vi "test_add_errors.vi"() -> ()   [LabVIEW 2020]
uses:
  <vilib>/Utility/miscctls.llb/LVPointTypeDef.ctl
panel:
  out "error out":errorcluster
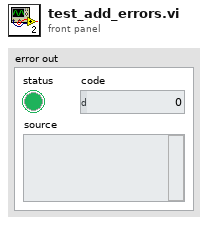
[diagram p1: front panel]
types:
  T1 = typedef "LVPointTypeDef.ctl" = cluster{"Horizontal":i16, "Vertical":i16}
  T2 = enum32{"invalid VI type", "Standard VI", "Control VI", "Global VI", "Polymorphic VI", "Configuration VI", "SubSystem", "Facade VI", "Method VI", "Statechart Diagram VI"}
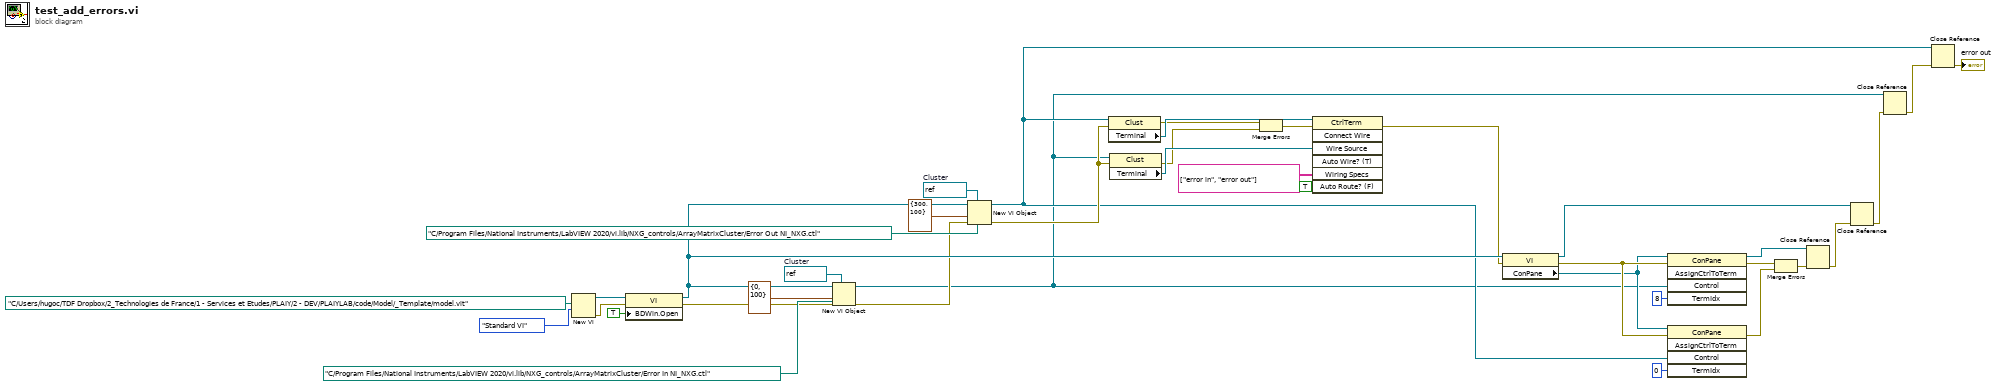
[diagram p0: block diagram]
diagram:
  w27 = refnum<vi> refnum  # Cluster
  w34 = refnum<vi> refnum  # Cluster
  n1 = New VI(9:T2."Standard VI" ("vi type (standard vi)"), 10:path "C:/Users/hugoc/TDF Dropbox/2_Technologies de France/1 - Services et Etudes/PLAIY/2 - DEV/PLAIYLAB/code/Model/_Template/model.vit" ("template")) -> (0:w36:errorcluster, 3:w30:refnum<vi>)  [unwired: 5 in]
  n2 = property class="VI"(reference=w30, error in=w36, "BDWin.Open"=TRUE ("Block Diagram Window:Open")) -> (reference out=w28:refnum<vi>, error out=w31:errorcluster)
  n3 = New VI Object(vi object class=w34, owner refnum=w28, position/next to=T1 {"Horizontal"=0, "Vertical"=100} ("location"), 6:path "C:/Program Files/National Instruments/LabVIEW 2020/vi.lib/NXG_controls/ArrayMatrixCluster/Error In NI_NXG.ctl" ("path"), 8:w31) -> (object refnum=w4:refnum<vi>, 0:w23:errorcluster)  [unwired: 3 in]
  n4 = New VI Object(vi object class=w27, owner refnum=w28, position/next to=T1 {"Horizontal"=300, "Vertical"=100} ("location"), 6:path "C:/Program Files/National Instruments/LabVIEW 2020/vi.lib/NXG_controls/ArrayMatrixCluster/Error Out NI_NXG.ctl" ("path"), 8:w23) -> (object refnum=w5:refnum<vi>, 0:w15:errorcluster)  [unwired: 3 in]
  n5 = property class="Clust"(reference=w5, error in=w15) -> (error out=w13:errorcluster, "Terminal"=w18:refnum<vi>)  [unwired: 1 out]
  n6 = property class="Clust"(reference=w4, error in=w15) -> (error out=w12:errorcluster, "Terminal"=w17:refnum<vi>)  [unwired: 1 out]
  n7 = Merge Errors(w13, w12) -> (w14:errorcluster)
  n8 = invoke class="CtrlTerm" method="Connect Wire"(reference=w18, error in=w14, "Wire Source"=w17, "Wiring Specs"=string[][] [["error in", "error out"]], "Auto Route? (F)"=TRUE) -> (error out=w10:errorcluster)  [unwired: 2 in, 6 out]
  n9 = property class="VI"(reference=w28, error in=w10) -> (reference out=w7:refnum<vi>, error out=w22:errorcluster, "ConPane"=w19:refnum<vi>)
  n10 = invoke class="ConPane" method="AssignCtrlToTerm"(reference=w19, error in=w22, "Control"=w4, "TermIdx"=u32 8 ("Terminal Index")) -> (reference out=w9:refnum<vi>, error out=w21:errorcluster)  [unwired: 1 in, 3 out]
  n11 = invoke class="ConPane" method="AssignCtrlToTerm"(reference=w19, error in=w22, "Control"=w5, "TermIdx"=u32 0 ("Terminal Index")) -> (error out=w20:errorcluster)  [unwired: 1 in, 4 out]
  n12 = Merge Errors(w21, w20) -> (w8:errorcluster)
  n13 = Close Reference(reference=w9, error in (no error)=w8) -> (error out=w6:errorcluster)
  n14 = Close Reference(reference=w7, error in (no error)=w6) -> (error out=w3:errorcluster)
  n15 = Close Reference(reference=w4, error in (no error)=w3) -> (error out=w2:errorcluster)
  n16 = Close Reference(reference=w5, error in (no error)=w2) -> (error out=→"error out":errorcluster)
